vi "Zero.vi"(8 "Zero":bool, 10 "Current Angle":dbl, 11 "Offset":dbl) -> (3 "Offset":dbl)   [LabVIEW 2013]
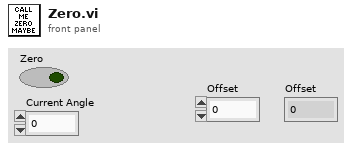
[diagram p1: front panel]
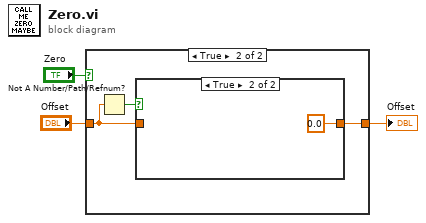
[diagram p0: block diagram]
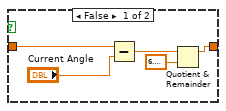
[diagram p3: hidden frame]
diagram:
  n1 = case shown="True" "Zero" {
    tunnel: "Offset" -> [w4 w6]
    tunnel: [w4 w5] -> w1
    frame False {
    }
    frame True {
      n2 = Not A Number/Path/Refnum?(number/path/refnum=w6) -> (NaN/Path/Refnum?=w7:bool)
      n3 = case shown="True" w7 {
        tunnel: w6 -> [w12 _]
        tunnel: [w9 0.0] -> w5
        frame False {
          n4 = Subtract(x=w12, y="Current Angle") -> (x-y=w10:dbl)
          n5 = Quotient & Remainder(x=w10, y=6.283185307179586) -> (x-y*floor(x/y)=w9:dbl)  [unwired: 1 out]
        }
        frame True {
        }
      }
    }
  }
  "Offset" <- w1
